vi "Guide_error_histo.vi"(0 "X Array":dbl[](array[numeric]), 1 "intervals":i32=10, 2 "Y array":dbl[](array[numeric]), 3 "limite haute":dbl=5.0, 6 "limite basse":dbl=-5.0) -> (4 "XY graph":cluster{dbl[], dbl[]}[](graph), 5 "RMS":dbl)   [LabVIEW 2019]
uses:
  <vilib>/Analysis/5stat.llb/RMS (DBL).vi
  Polymorphics/Distance(array).vi
  <vilib>/Analysis/NI_AALBase.lvlib
  <vilib>/Analysis/NI_AALPro.lvlib
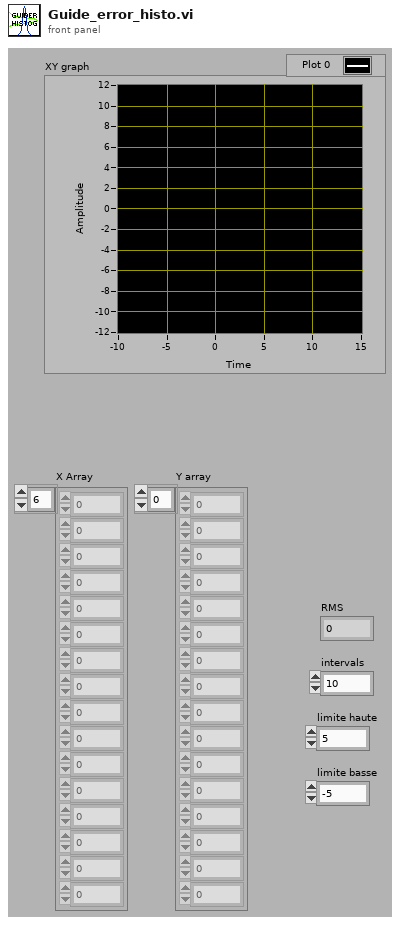
[diagram p1: front panel]
types:
  T1 = cluster{"normailzed array 2":dbl[], "X Values":dbl[]}
  T2 = cluster{"X Values":dbl[], "normailzed array 2":dbl[]}
  T3 = cluster{"normailzed array 2":dbl[], "X Values":dbl[]}[]
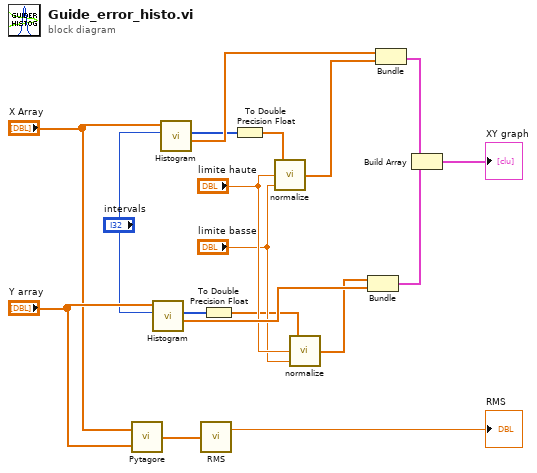
[diagram p0: block diagram]
diagram:
  n1 = call-poly "Pytagore.vi"("Y"="Y array", "X"="X Array") -> ("Dist"=w10:dbl[])
  n2 = call <vilib>:"Histogram.vi"("intervals"="intervals", "X"="Y array") -> ("X Values"=w16:dbl[], "Histogram: h(x)"=w13:i32[])  [unwired: 6 in, 2 out]
  n3 = call <vilib>:"Histogram.vi"("intervals"="intervals", "X"="X Array") -> ("X Values"=w15:dbl[], "Histogram: h(x)"=w14:i32[])  [unwired: 6 in, 2 out]
  n4 = call-poly <vilib>:"RMS.vi"("X"=w10) -> ("rms value"=→"RMS":dbl)  [unwired: 1 out]
  n5 = To Double Precision Float(number=w13) -> (double precision float=w1:dbl[])
  n6 = To Double Precision Float(number=w14) -> (double precision float=w2:dbl[])
  n7 = call "normalize.vi"("limite basse"="limite basse", "limite haute"="limite haute", "Input Array"=w2) -> ("normailzed array 2"=w11:dbl[])
  n8 = call "normalize.vi"("limite basse"="limite basse", "limite haute"="limite haute", "Input Array"=w1) -> ("normailzed array 2"=w12:dbl[])
  n9 = Bundle("normailzed array 2"=w12, "X Values"=w16) -> (w18:T1)  [unwired: 1 in]
  n10 = Bundle("X Values"=w15, "normailzed array 2"=w11) -> (w17:T2)  [unwired: 1 in]
  n11 = Build Array(w17, w18) -> (→"XY graph":T3)
